vi "MIL CEL Reading.vi"(7 "ENUM":T1=enum."CLOSE", 8 "error in (no error)":errorcluster) -> (0 "error out":errorcluster, 2 "data":dbl[](array[numeric]) format="%.2f")   [LabVIEW 2025]
uses:
  Controls/CAN READ ENUM.ctl
  Application/Common VIs/Read File Data.ctl
  <vilib>/xnet/xnet.llb/XNET Create Session (Signal Input Single-point).vi
  <vilib>/xnet/xnet.llb/XNET Read (Signal Single-point).vi
panel:
  out "session out 2":refnum<k21>
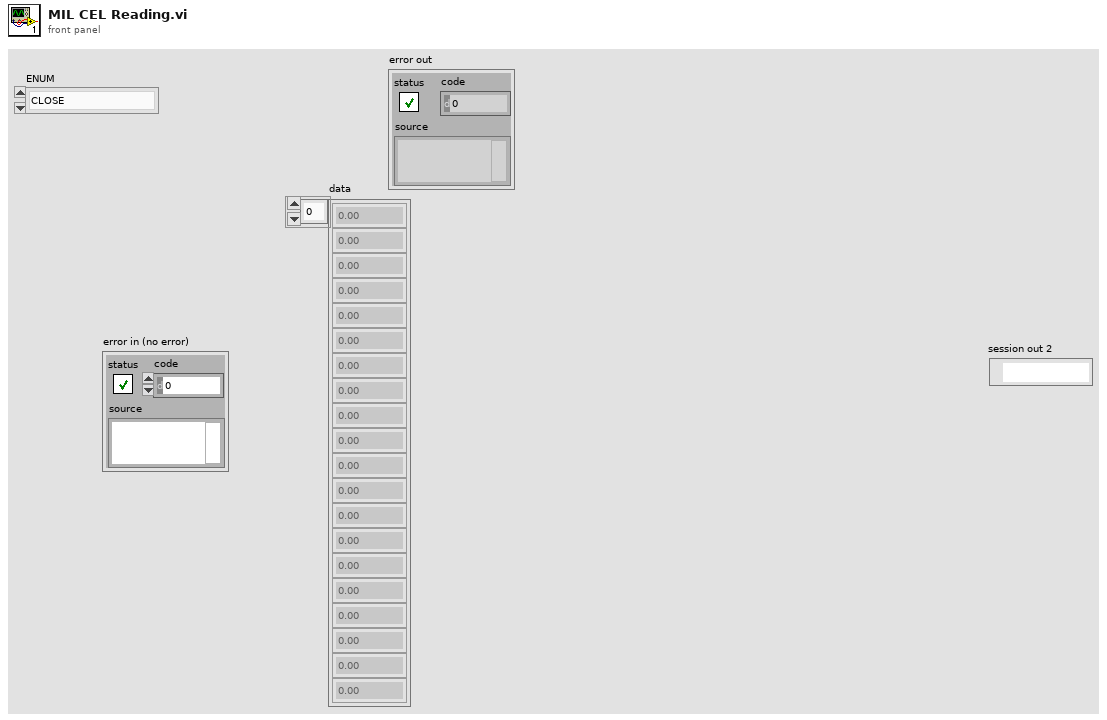
[diagram p1: front panel]
types:
  T1 = typedef "CAN READ ENUM.ctl" = enum16{"OPEN", "READ", "CLOSE"}
  T2 = typedef "Read File Data.ctl" = enum16{"Get Data", "Set Data"}
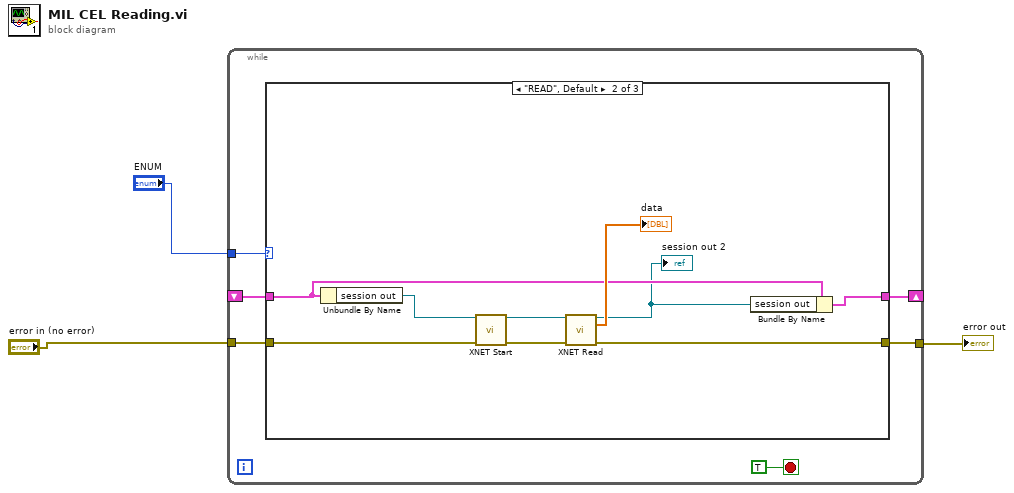
[diagram p0: block diagram]
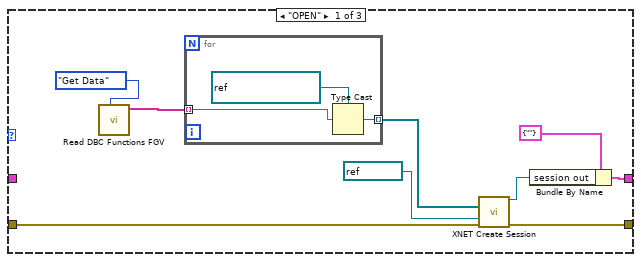
[diagram p2: hidden frame]
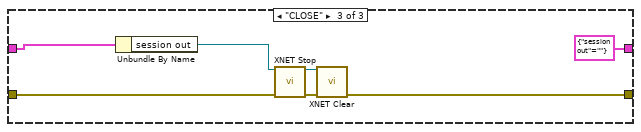
[diagram p3: hidden frame]
diagram:
  n1 = while {
    tunnel: "ENUM" -> [w8]
    tunnel: "error in (no error)" -> [w7]
    tunnel: [w6] -> w1
    shift-right: [w5] -> _
    shift-left: _ -> [w4]
    stop <- TRUE stop-if-true
    n2 = case shown="\"READ\", Default" w8 {
      tunnel: w7 -> [w14 w27 w35]
      tunnel: [w13 w22 w32] -> w6
      tunnel: [w10 w23 cluster{"session out":refnum<k21>} {"session out"=""}] -> w5
      tunnel: w4 -> [_ w25 w34]
      frame "OPEN" {
        n3 = call "Read DBC Functions FGV.vi"("Enum"=Read_File_Data."Get Data") -> ("DBC FUNCTIONS OUT"=w17:string[])  [unwired: 9 in, 1 out]
        n4 = for {
          tunnel: w17 -> [w20] mode=indexing
          tunnel: [w19] -> w18 mode=indexing
          n5 = Type Cast(type=refnum<k21> "EngineOilPrLamp\nTEST" ("XNET Signal"), x=w20) -> (*(type *) &x=w19:refnum<k21>)
        }
        n6 = call-poly <vilib>:"XNET Create Session.vi"("signal list"=w18, "interface"=refnum<k21> "CAN1" ("Select Interface"), "error in (no error)"=w14) -> ("session out"=w11:refnum<k21>, "error out"=w13:errorcluster)  [unwired: 11 out]
        n7 = Bundle By Name(cluster=cluster{"session out":refnum<k21>} {"session out"=""}, "session out"=w11) -> (w10:cluster{"session out":refnum<k21>})
      }
      frame "READ", Default {
        n8 = Unbundle By Name(w25) -> ("session out"=w26:refnum<k21>)
        n9 = call <vilib>:"XNET Start.vi"("session in"=w26, "error in (no error)"=w27) -> ("session out"=w28:refnum<k21>, "error out"=w29:errorcluster)  [unwired: 12 in]
        n10 = call-poly <vilib>:"XNET Read.vi"("session in"=w28, "error in (no error)"=w29) -> ("session out"=w24:refnum<k21>, "data"=→"data":dbl[], "error out"=w22:errorcluster)  [unwired: 11 in]
        "session out 2" <- w24
        n11 = Bundle By Name(cluster=w25, "session out"=w24) -> (w23:cluster{"session out":refnum<k21>})
      }
      frame "CLOSE" {
        n12 = Unbundle By Name(w34) -> ("session out"=w33:refnum<k21>)
        n13 = call <vilib>:"XNET Stop.vi"("session in"=w33, "error in (no error)"=w35) -> ("session out"=w36:refnum<k21>, "error out"=w37:errorcluster)  [unwired: 12 in]
        n14 = call <vilib>:"XNET Clear.vi"("session in"=w36, "error in (no error)"=w37) -> ("error out"=w32:errorcluster)  [unwired: 13 in]
      }
    }
  }
  "error out" <- w1
